vi "Set Front Panel TestSuite Object Control Value.vi"(8 "error in":errorcluster, 10 "Control (F: Indicator)":bool=TRUE, 11 "vi reference":refnum<vi>) -> (0 "error out":errorcluster, 1 "Found?":bool, 2 "Control Value":T1, 3 "dup vi reference":refnum<vi>)   [LabVIEW 2013, in "VITesterUtilities.lvlib"]
doc: "Sets the FP control value of an LVClass control, whose type matches the specific type of object in <B>Object in</B> to the value of <B>Object in</B>."
uses:
  Libraries/VITesterUtilities.lvlib
  Classes/TestSuite/TestSuite.lvclass
  JKI Reuse/Is an Error (error cluster)__jki_lib_error_handling -- VI Tester.vi
panel:
  # "Copyright © 2007 James Kring, Inc. All rights reserved.\n\nAuthor: Jim Kring <jim.kring@jameskring.com>\n\nThis library is provided \"AS IS\" , WITHOUT WARRANTIES OR \nCONDITIONS OF ANY KIND, either express or implied.\n\nJames Kring, Inc. -- http://www.jameskring.com"
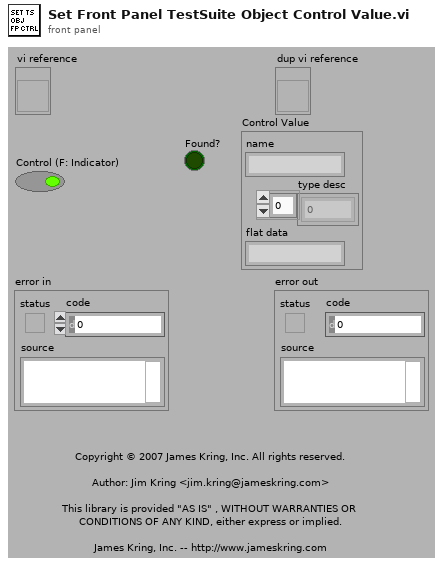
[diagram p1: front panel]
types:
  T1 = cluster{"name":string, "type desc":i16[], "flat data":string}
  T2 = cluster{"name":string, "type desc":i16[], "flat data":string}[]
  T3 = typedef "Type Descriptor Header__ogtk.ctl" = cluster{"length":u16, "private":u8, "type":T4, "# elements":u16}
  T4 = typedef "Type Descriptor Enumeration__ogtk.ctl" = enum8{"<Null>", "I8", "I16", "I32", "I64", "U8", "U16", "U32", "U64", "SGL", "DBL", "EXT", "CSG", "CDB", "CXT", "0x0F", "0x10", "0x11", "0x12", "0x13", "0x14", "Enum U8", "Enum U16", "Enum U32", "Enum U64", "SGL PQ", "DBL PQ", "EXT PQ", "CSG PQ", "CDB PQ", "CXT PQ", "0x1F", "0x20", "Boolean", "0x22", "0x23", "0x24", "0x25", "0x26", "0x27", "0x28", "0x29", "0x2A", "0x2B", "0x2C", "0x2D", "0x2E", "0x2F", "String", "0x31", "Path", "Pict", "0x34", "0x35", "0x36", "DAQ", "0x38", "0x39", "0x3A", "0x3B", "0x3C", "0x3D", "0x3E", "0x3F", "Array", "0x41", "0x42", "0x43", "0x44", "0x45", "0x46", "0x47", "0x48", "0x49", "0x4A", "0x4B", "0x4C", "0x4D", "0x4E", "0x4F", "Cluster", "0x51", "0x52", "Variant", "Waveform", "0x55", "0x56", "0x57", "0x58", "0x59", "0x5A", "0x5B", "0x5C", "0x5D", "0x5E", "0x5F", "0x60", "0x61", "0x62", "0x63", "0x64", "0x65", "0x66", "0x67", "0x68", "0x69", "0x6A", "0x6B", "0x6C", "0x6D", "0x6E", "0x6F", "Refnum"}
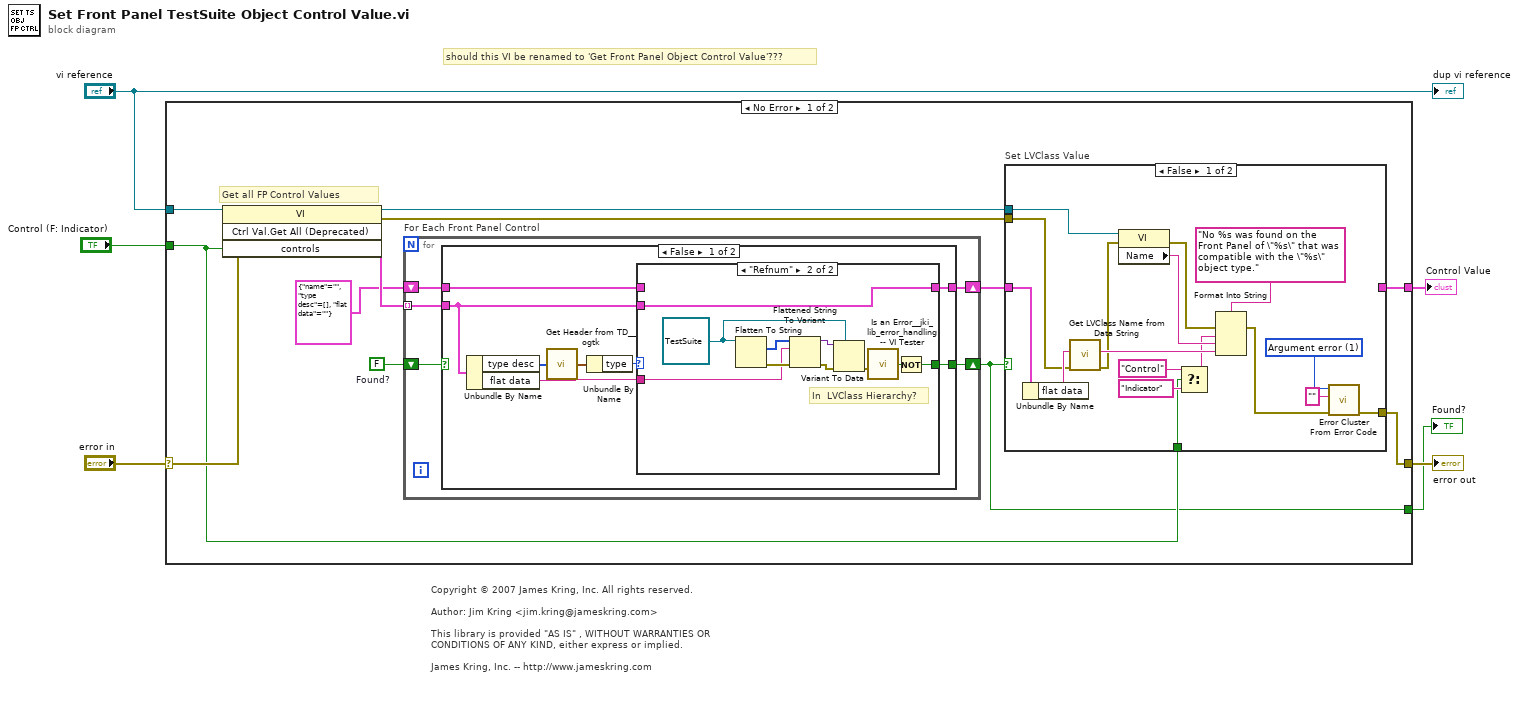
[diagram p0: block diagram]
diagram:
  # "should this VI be renamed to 'Get Front Panel Object Control Value'???"
  # "Copyright © 2007 James Kring, Inc. All rights reserved.\n\nAuthor: Jim Kring <jim.kring@jameskring.com>\n\nThis library is provided \"AS IS\" , WITHOUT WARRANTIES OR \nCONDITIONS OF ANY KIND, either express or implied.\n\nJames Kring, Inc. -- http://www.jameskring.com"
  n1 = case shown="No Error" "error in" {
    selector: "error in" -> [w12 w64]
    tunnel: [w18 w64] -> w5
    tunnel: "vi reference" -> [w16 _]
    tunnel: "Control (F: Indicator)" -> [w9 _]
    tunnel: [w8 _] -> w2
    tunnel: [w7 _] -> w1
    frame No Error {
      w13 = FALSE  # Found?
      # "Get all FP Control Values"
      n2 = invoke class="VI" method="Ctrl Val.Get All (Deprecated)"(reference=w16, error in=w12, "controls"=w9) -> (reference out=w17:refnum<vi>, error out=w15:errorcluster, "Get All Control Values"=w14:T2)  [unwired: 1 in, 1 out]
      n3 = for "For Each Front Panel Control" {
        tunnel: w14 -> [w22] mode=indexing
        shift-right: [w23] -> w7
        shift-left: w13 -> [w21]
        shift-right: [w20] -> w11
        shift-left: T1 {"name"="", "type desc"=[], "flat data"=""} -> [w19]
        n4 = case shown="False" w21 {
          selector: w21 -> [_ w44]
          tunnel: [w27 w44] -> w23
          tunnel: w22 -> [w26 _]
          tunnel: [w25 w43] -> w20
          tunnel: w19 -> [w24 w43]
          frame False {
            n5 = Unbundle By Name(w26) -> ("type desc"=w31:i16[], "flat data"=w28:string)
            n6 = call <userlib>:"Get Header from TD__ogtk.vi"("Type Descriptor"=w31) -> ("Type Descriptor Header"=w30:T3)
            n7 = Unbundle By Name(w30) -> ("type"=w29:T4)
            n8 = case shown="\"Refnum\"" w29 {
              tunnel: w28 -> [_ w35]
              tunnel: [_ w41] -> w27
              tunnel: w26 -> [_ w34]
              tunnel: [w32 w34] -> w25
              tunnel: w24 -> [w32 _]
              frame Default {
              }
              frame "Refnum" {
                w33 = refnum<class "TestSuite.lvclass"> refnum ("reference in")
                # "In  LVClass Hierarchy?"
                n9 = Flatten To String(anything=w33) -> (type string=w40:i16[], error out=w38:errorcluster)  [unwired: 3 in, 1 out]
                n10 = Flattened String To Variant(4:w38, 6:w35, 7:w40) -> (0:w37:errorcluster, 3:w39:variant)
                n11 = Variant To Data(error in=w37, type=w33, Variant=w39) -> (error out=w36:errorcluster)  [unwired: 1 out]
                n12 = call-poly "Is an Error__jki_lib_error_handling -- VI Tester.vi"("error in"=w36) -> ("error?"=w42:bool)  [unwired: 8 in]
                n13 = Not(x=w42) -> (.not. x?=w41:bool)
              }
            }
          }
          frame True {
          }
        }
      }
      n14 = case "Set LVClass Value" shown="False" w7 {
        tunnel: w11 -> [w53 w63]
        tunnel: [w61 w62] -> w18
        tunnel: w17 -> [w58 _]
        tunnel: w15 -> [w50 w62]
        tunnel: w9 -> [w45 _]
        tunnel: [_ w63] -> w8
        frame False {
          w60 = 1 items=["No error", "Argument error", "Memory is full", "Out of zone", "End of file", "File already open", "Generic file I/O error", "File not found", "File permission error", "Disk is full", "Duplicate path", "Too many files open", "System feature not enabled", "Resource file not found", "Cannot add resource", "Resource not found", "Image not found", "Image memory error", "Pen does not exist", "Config type invalid", "Config token not found", "Config parse error", "Config memory error", "Bad external code format", "Bad external code offset", "External code not present", "Null window", "Destroy window error", "Null menu", "Print aborted", "Bad print record", "Print driver error", "Windows error during printing", "Memory error during printing", "Print dialog error", "Generic print error", "Invalid device refnum", "Device not found", "Device parameter error", "Device unit error", "Cannot open device", "Device call aborted", "Generic error", "Cancelled by user", "Object ID too low", "Object ID too high", "Object not in heap", "Unknown heap", "Unknown object (invalid DefProc)", "Unknown object (DefProc not in table)", "Message out of range", "Invalid (null) method", "Unknown message", "Manager call not supported", "Bad address", "Network operation in progress", "Network operation timed out", "Connection is busy", "Network attribute not supported", "Network error", "Address in use", "System out of memory", "Connection aborted", "Connection refused", "Not connected", "Already connected", "Connection closed", "Initialization error (interapplication manager)", "Bad occurrence", "Wait on unbound occurrence handler", "Occurrence queue overflow", "Datalog type conflict", "Unused", "Unrecognized type (interapplication manager)", "Memory corrupt", "Failed to make temporary DLL", "Old CIN version", "Drag socket not found", "Failed to load drop-object", "Failed to register OLE object", "Failed to release OLE object", "Format specifier type mismatch", "Unknown format specifier", "Too few format specifiers", "Too many format specifiers", "Scan failed", "Newer CIN version", "Error converting to variant", "Runtime menu error", "Password tampered", "Variant attribute not found", "Incompatible variant data type", "Event data is not available", "Event Store is not present", "Occurrence is not found", "Event Queue is not created", "Event info is not available", "Refnum passed is NULL", "Error retrieving Class GUID", "Error retrieving CoClass GUID", "Error retrieving TypeLib GUID.", "Bad built application magic bytes.", "Specific driver is different from the specific driver associated with the Logical Name.", "There is no session opened to the class driver.", "Max Error", "MAX - Error with config objects", "MAX - Error loading configuration", "MAX - Group not supported"]
          n15 = Unbundle By Name(w53) -> ("flat data"=w52:string)
          n16 = call "Get LVClass Name from Data String.vi"("error in"=w50, "LVClass Data String"=w52) -> ("error out"=w49:errorcluster, "LVClass Name"=w51:string)  [unwired: 8 in]
          n17 = property class="VI"(reference=w58, error in=w49) -> (error out=w55:errorcluster, "Name"=w57:string)  [unwired: 1 out]
          n18 = Select(t="Control", s=w45, f="Indicator") -> (s? t:f=w48:string)
          n19 = Format Into String(format string="No %s was found on the Front Panel of \"%s\" that was compatible with the \"%s\" object type.", error in=w55, w48, w57, w51) -> (error out=w54:errorcluster)  [unwired: 1 in, 1 out]
          n20 = call <vilib>:"Error Cluster From Error Code.vi"("error in (no error)"=w54, "error message (\"\")"="" ("error message (\"\")"), "error code (0)"=w60) -> ("error out"=w61:errorcluster)  [unwired: 6 in]
        }
        frame True {
        }
      }
    }
    frame Error {
    }
  }
  "error out" <- w5
  "Control Value" <- w2
  "Found?" <- w1
  "dup vi reference" <- "vi reference"
